vi "user actions.vi"(8 "error in":errorcluster, 9 "Amount":string, 10 "user action":T3, 11 "all data in":T1) -> (0 "error out":errorcluster, 1 "Message":string, 2 "result":string, 3 "all data out":T1)   [LabVIEW 2015]
uses:
  all data.ctl
  User data.ctl
  user action.ctl
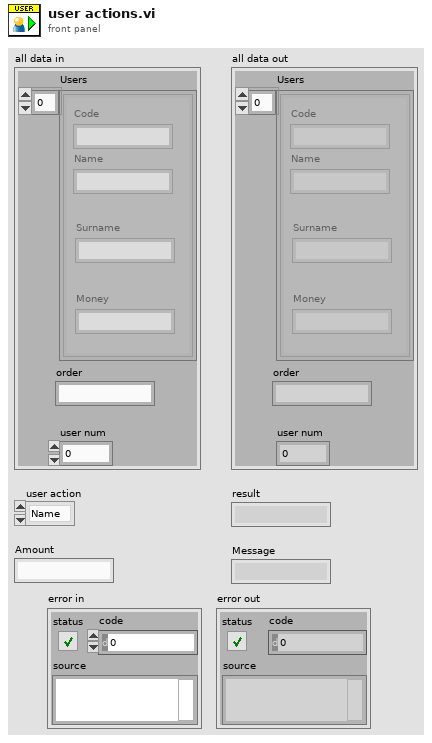
[diagram p1: front panel]
types:
  T1 = typedef "all data.ctl" = cluster{"order":string, "Users":T2[], "user num":i32}
  T2 = typedef "User data.ctl" = cluster{"Code":string, "Name":string, "Surname":string, "Money":string}
  T3 = typedef "user action.ctl" = enum16{"Name", "Withdraw", "Deposit", "Balance"}
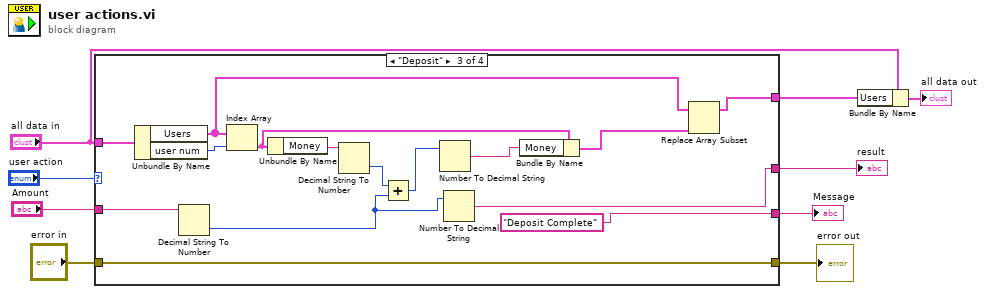
[diagram p0: block diagram]
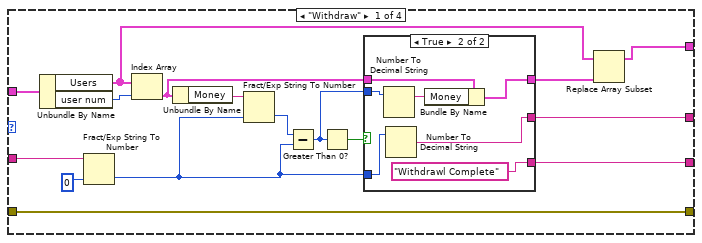
[diagram p2: hidden frame]
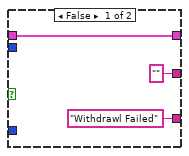
[diagram p3: hidden frame]
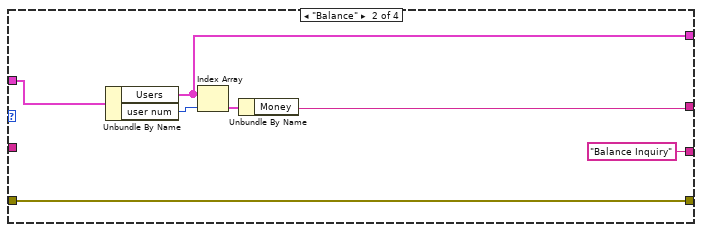
[diagram p4: hidden frame]
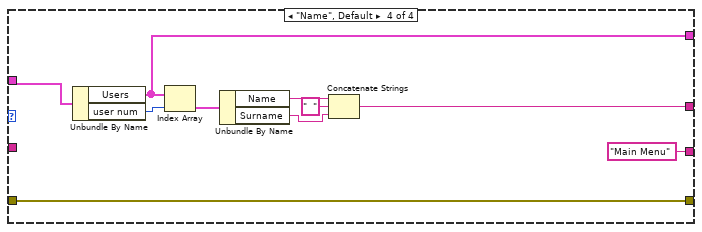
[diagram p5: hidden frame]
diagram:
  n1 = case shown="\"Deposit\"" "user action" {
    tunnel: "all data in" -> [w24 w40 w49 w67]
    tunnel: [w14 w39 w43 w61] -> w3
    tunnel: "Amount" -> [w22 _ w50 _]
    tunnel: [w15 w36 w48 w60] -> w7
    tunnel: [w13 "Balance Inquiry" ("Message") "Deposit Complete" ("Message") "Main Menu" ("Message")] -> w8
    tunnel: "error in" -> [w12 w37 w46 w58]
    tunnel: [w12 w37 w46 w58] -> w1
    frame "Withdraw" {
      n2 = Unbundle By Name(w24) -> ("Users"=w17:T2[], "user num"=w25:i32)
      n3 = Fract/Exp String To Number(string=w22, default (0 dbl)=0) -> (number=w10:i32)  [unwired: 2 in, 1 out]
      n4 = Index Array(array=w17, index=w25) -> (element=w18:T2)
      n5 = Unbundle By Name(w18) -> ("Money"=w23:string)
      n6 = Fract/Exp String To Number(string=w23, default (0 dbl)=w10) -> (number=w21:i32)  [unwired: 2 in, 1 out]
      n7 = Subtract(x=w21, y=w10) -> (x-y=w19:i32)
      n8 = Greater Than 0?(x=w19) -> (x > 0?=w20:bool)
      n9 = case shown="True" w20 {
        tunnel: w18 -> [w28 w35]
        tunnel: w19 -> [_ w34]
        tunnel: [w28 w33] -> w16
        tunnel: ["" w29] -> w14
        tunnel: ["Withdrawl Failed" ("Message") "Withdrawl Complete" ("Message")] -> w13
        tunnel: w10 -> [_ w30]
        frame False {
        }
        frame True {
          n10 = Number To Decimal String(number=w34) -> (decimal integer string=w32:string)  [unwired: 1 in]
          n11 = Number To Decimal String(number=w30) -> (decimal integer string=w29:string)  [unwired: 1 in]
          n12 = Bundle By Name(cluster=w35, "Money"=w32) -> (w33:T2)
        }
      }
      n13 = Replace Array Subset(array=w17, new element=w16) -> (w15:T2[])  [unwired: 1 in]
    }
    frame "Balance" {
      n14 = Unbundle By Name(w40) -> ("Users"=w36:T2[], "user num"=w41:i32)
      n15 = Index Array(array=w36, index=w41) -> (element=w42:T2)
      n16 = Unbundle By Name(w42) -> ("Money"=w39:string)
    }
    frame "Deposit" {
      n17 = Unbundle By Name(w49) -> ("Users"=w56:T2[], "user num"=w51:i32)
      n18 = Decimal String To Number(string=w50) -> (number=w44:i32)  [unwired: 2 in, 1 out]
      n19 = Index Array(array=w56, index=w51) -> (element=w55:T2)
      n20 = Unbundle By Name(w55) -> ("Money"=w52:string)
      n21 = Decimal String To Number(string=w52) -> (number=w53:i32)  [unwired: 2 in, 1 out]
      n22 = Add(x=w53, y=w44) -> (x+y=w54:i32)
      n23 = Number To Decimal String(number=w54) -> (decimal integer string=w45:string)  [unwired: 1 in]
      n24 = Number To Decimal String(number=w44) -> (decimal integer string=w43:string)  [unwired: 1 in]
      n25 = Bundle By Name(cluster=w55, "Money"=w45) -> (w57:T2)
      n26 = Replace Array Subset(array=w56, new element=w57) -> (w48:T2[])  [unwired: 1 in]
    }
    frame "Name", Default {
      n27 = Unbundle By Name(w67) -> ("Users"=w60:T2[], "user num"=w66:i32)
      n28 = Index Array(array=w60, index=w66) -> (element=w65:T2)
      n29 = Unbundle By Name(w65) -> ("Name"=w64:string, "Surname"=w62:string)
      n30 = Concatenate Strings(w64, "  " ("string"), w62) -> (w61:string)
    }
  }
  "result" <- w3
  "Message" <- w8
  "error out" <- w1
  n31 = Bundle By Name(cluster="all data in", "Users"=w7) -> (→"all data out":T1)
